vi "WILT Individual Plots.vi"(0 "File Name":T1, 1 "Station Data":T3 {"Night Cycle Count" format="%04d"; "Day Cycle Count" format="%04d"}, 2 "GUI Aisle 1 (SLAT).":T3[](array[typedef]) {"Night Cycle Count" format="%04d"; "Day Cycle Count" format="%04d"}, 5 "Error In":errorcluster, 6 "Station Index":i32) -> (14 "GUI Output":T3[](array[typedef]) {"Night Cycle Count" format="%04d"; "Day Cycle Count" format="%04d"}, 15 "Station Data Out":T3 {"Night Cycle Count" format="%04d"; "Day Cycle Count" format="%04d"}, 19 "Error Out":errorcluster)   [LabVIEW 2016]
uses:
  Type Definitions/WILT Dryer.ctl
  Type Definitions/WILT Dryer Details.ctl
  Type Definitions/WILT Agilent Channel Definition.ctl
  Type Definitions/WILT DAQ Data.ctl
  Utility/Save File/File Setup (Public)/Type Definition/Save File DOE File Path Control.ctl
  Utility/Save File/File Setup (Public)/Type Definition/Save File DOE Data Save Filepaths.ctl
  Utility/Save File/File Setup.lvlib
panel:
  in  "OK":bool
  out "Label":string
  in  "Tab Control":enum32{"Plots", "File Names", "Debug"}(tab)
  out "Mixed Signal Graph":cluster{timestamp[], "all rows":dbl[]}[](graph)
  in  "Debug":bool
  out "Lab ID":string
  out "Dryer Details.TR Number":string
  out "Day Cycle Count 2":i32
  out "Night Cycle Count 2":i32
  in  "Night Cycle Count":i32
  in  "Day Cycle Count":i32
  in  "TR Number:":string
  in  "Lab ID:":string
  # "Model Information"
  # "Day"
  # "Night"
  # "Day"
  # "Night"
  # "Day"
  # "Night"
  # "Day"
  # "Night"
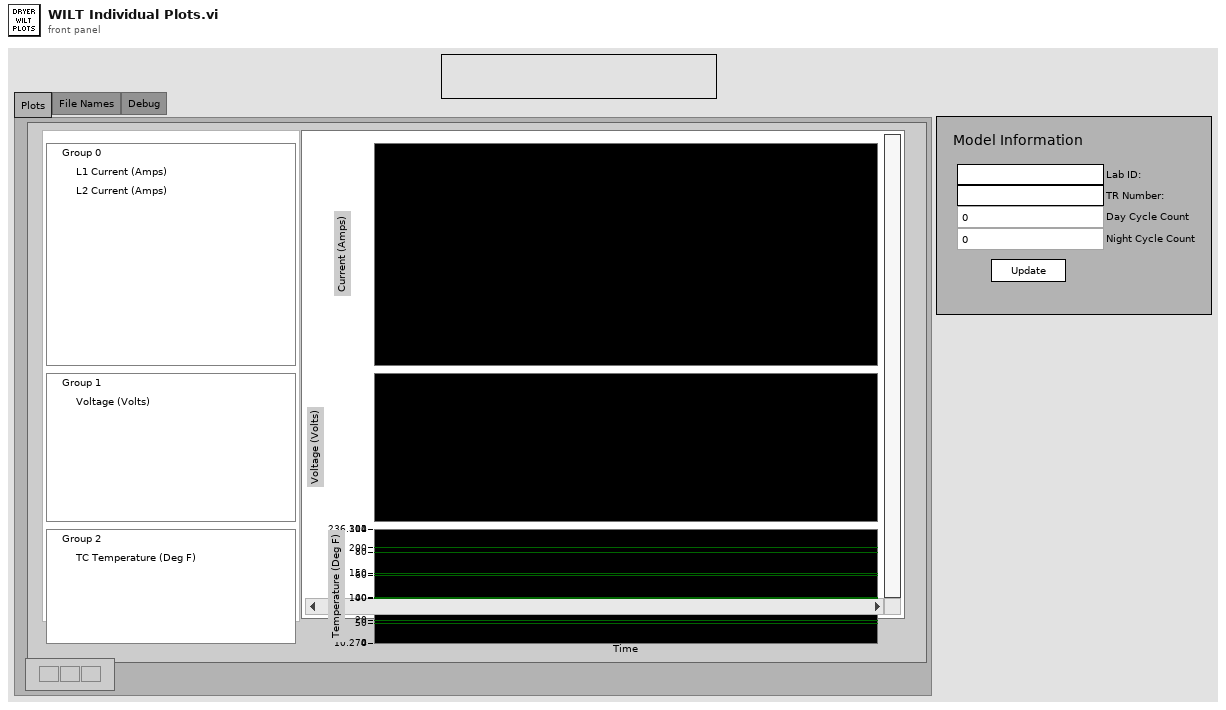
[diagram p1: front panel]
types:
  T1 = typedef "File Setup.lvlib/Save File DOE File Path Control.ctl" = cluster{"General Setup Paths":cluster{"Calibration File Path":path, "DOE Capacity Path":path, "Data Folder Path":path, "RLT Backup Data Path":path, "Tool Base Path":path, "General Startup Config Path":path, "File Save Previous Run Path":path, "File Save Configuration Data Path":path}, "Data File Paths":T2, "New Summary Created":bool, "Check Location Interval (Second)":i32}
  T2 = typedef "File Setup.lvlib/Save File DOE Data Save Filepaths.ctl" = cluster{"Data File Path":path, "Debug File Path":path, "Bus Log Path":path, "Current":path, "Summary":path}
  T3 = typedef "WILT Dryer.ctl" = cluster{"Lab ID":string, "Day Cycle Count":i32, "Station Label":string, "Dryer Details":T4, "Status Color":u32, "Invisible Button":bool, "Night Cycle Count":i32, "Station Index":i32, "Cycle Index":string, "Audit Alert":bool, "Agilent Channel Definition":T5, "DAQ Data":T6}
  T4 = typedef "WILT Dryer Details.ctl" = cluster{"Station":string, "Lab ID":string, "TR Number":string}
  T5 = typedef "WILT Agilent Channel Definition.ctl" = cluster{"Channel":string, "Station":string, "Label":string, "Agilent Station":string, "Data":dbl}
  T6 = typedef "WILT DAQ Data.ctl" = cluster{"L1 Current":dbl, "L2 Current":dbl, "Temperature  Deg F (TC)":dbl, "Volts":dbl, "Volts (208)":dbl, "SW (208)":dbl}
  T7 = enum32{"invalid app kind", "Development System", "Run Time System", "Student Edition", "Embedded LabVIEW", "Evaluation", "Custom"}
  T8 = enum32{"Invalid", "Standard", "Closed", "Hidden", "Minimized", "Maximized"}
  T9 = cluster{"Core":cluster{"Current VI Reference":refnum<vi>, "Close Panel on Exit?":bool}, "File Name":T1, "Station Data":T3, "GUI Aisle 1 (SLAT).":T3[]}
  T10 = cluster{"Current VI Reference":refnum<vi>, "Close Panel on Exit?":bool}
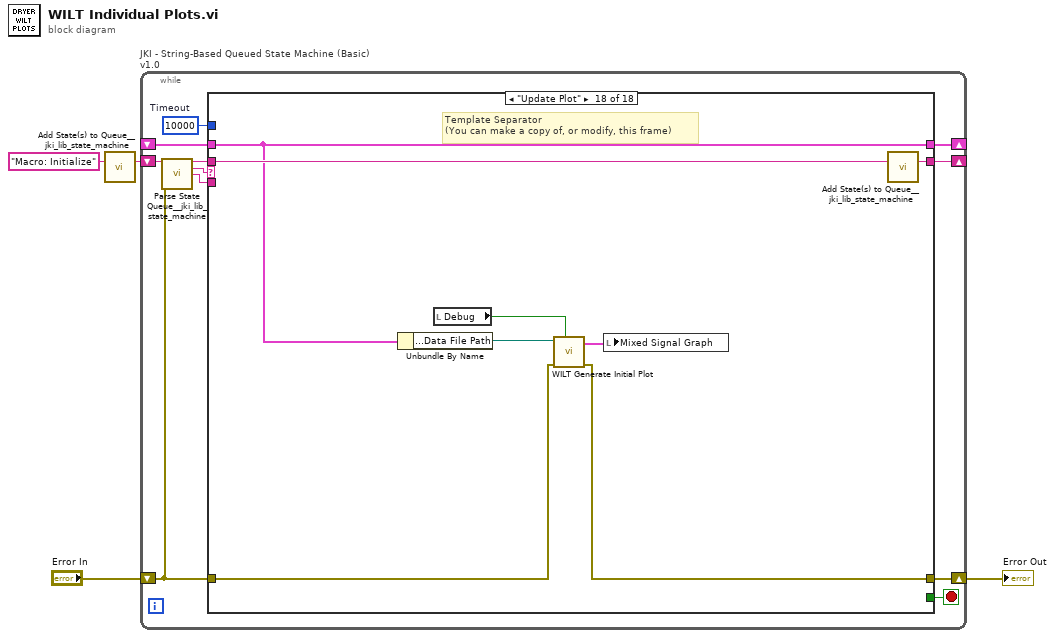
[diagram p0: block diagram]
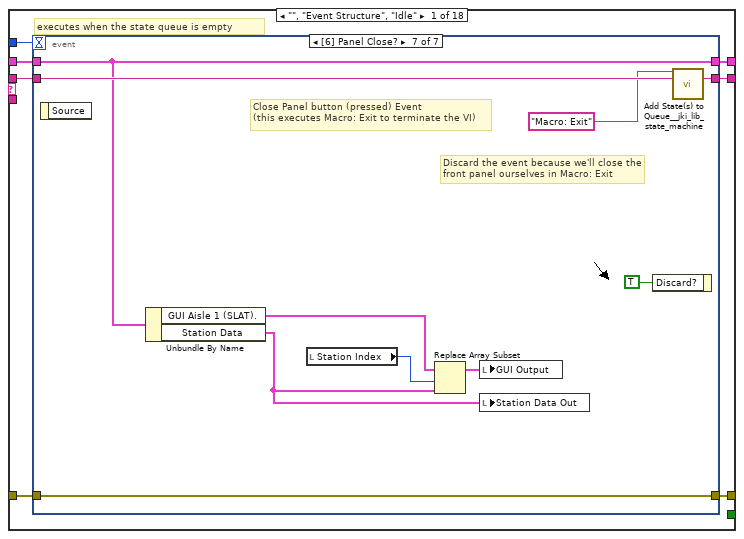
[diagram p2: hidden frame]
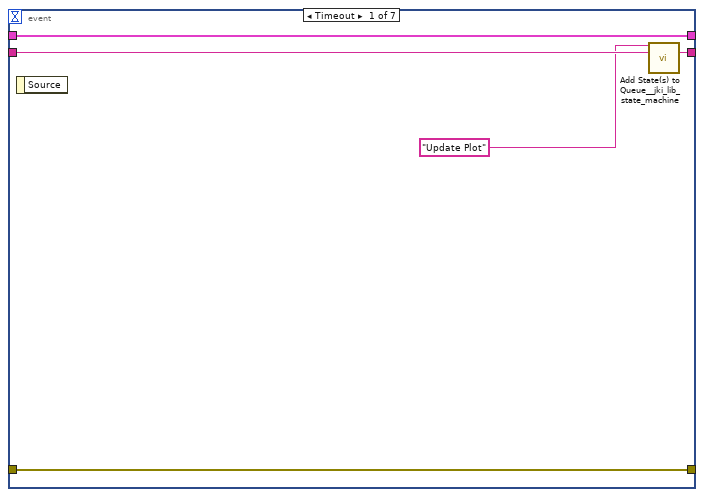
[diagram p3: hidden frame]
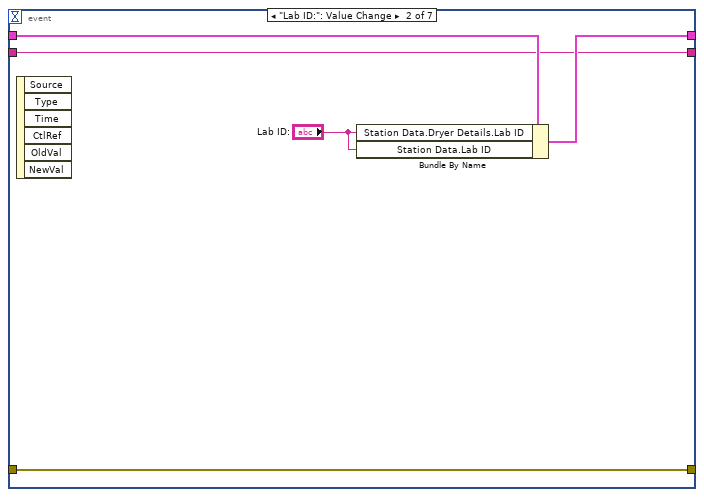
[diagram p4: hidden frame]
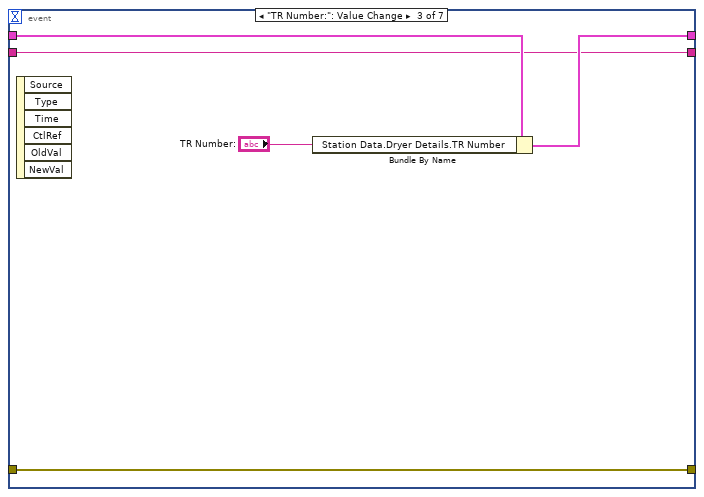
[diagram p5: hidden frame]
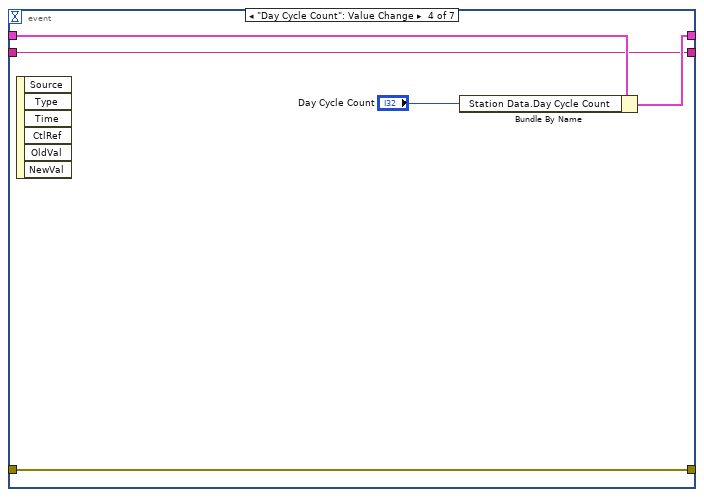
[diagram p6: hidden frame]
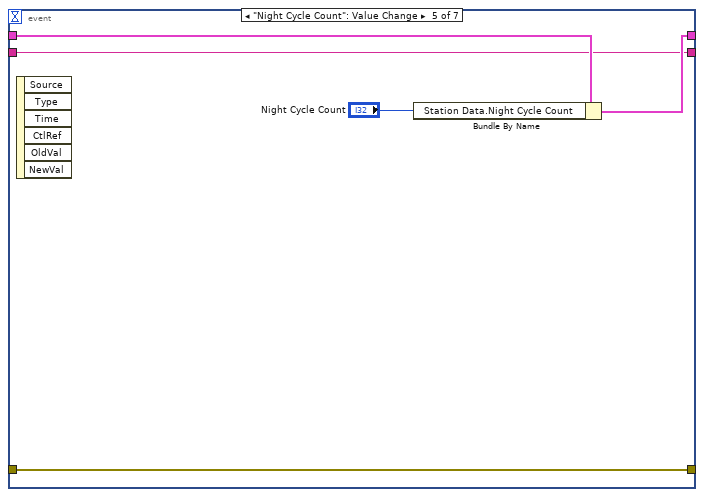
[diagram p7: hidden frame]
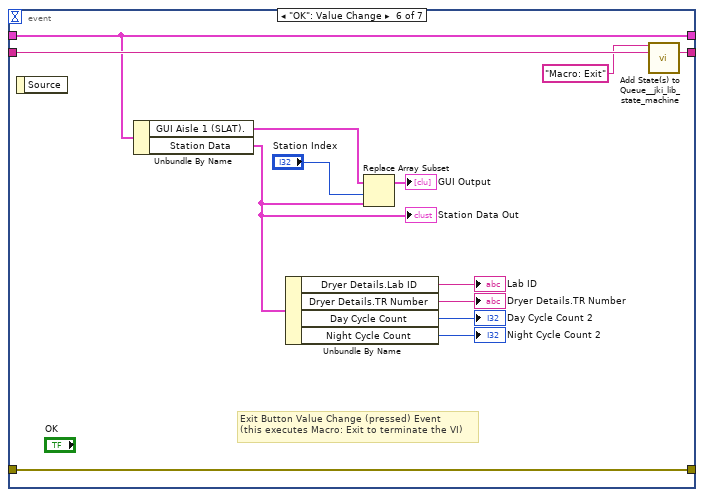
[diagram p8: hidden frame]
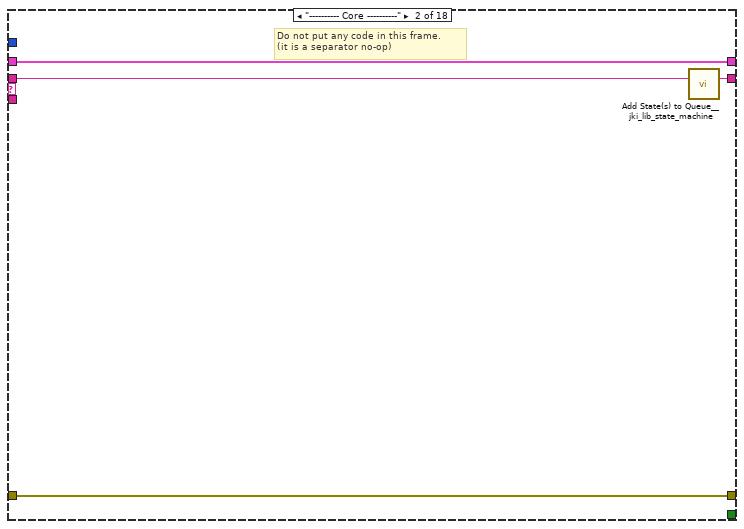
[diagram p9: hidden frame]
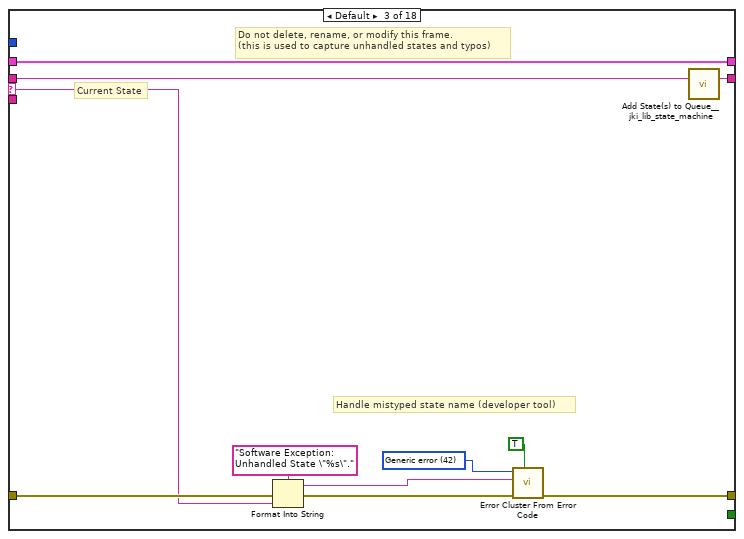
[diagram p10: hidden frame]
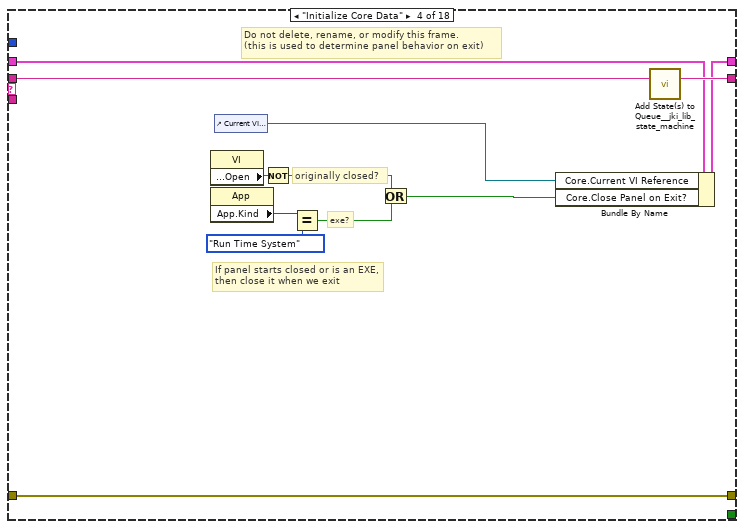
[diagram p11: hidden frame]
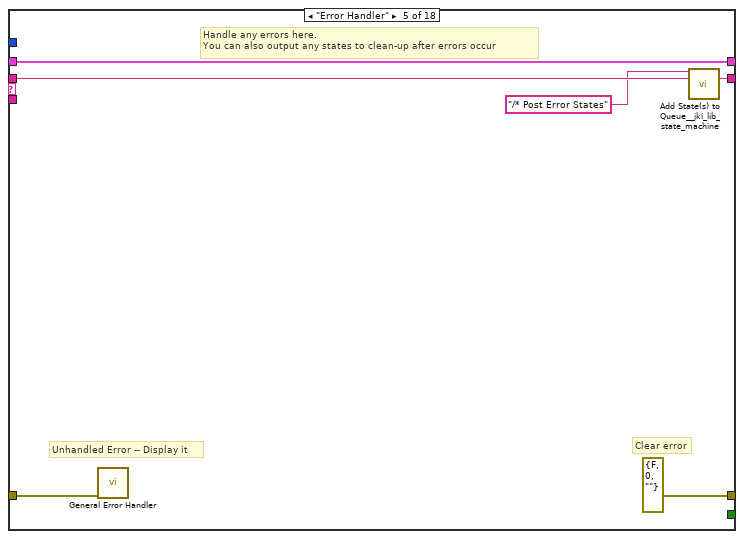
[diagram p12: hidden frame]
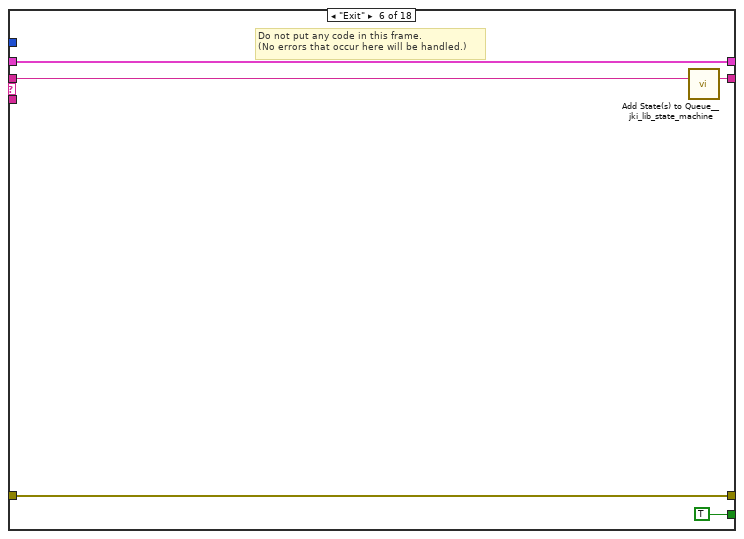
[diagram p13: hidden frame]
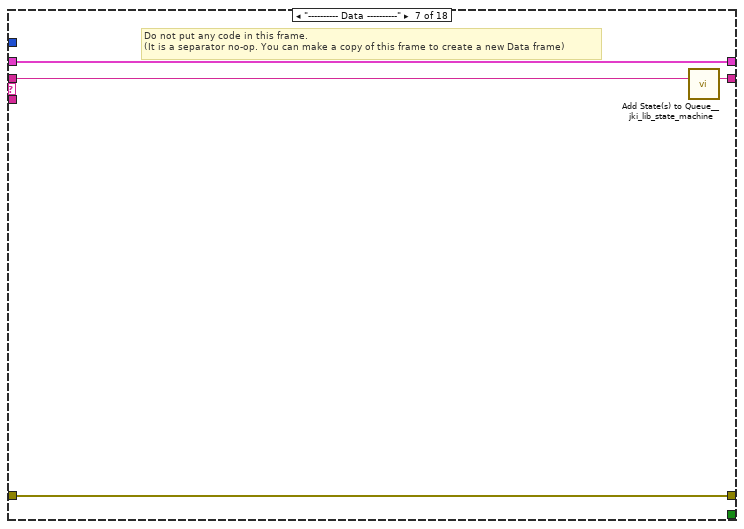
[diagram p14: hidden frame]
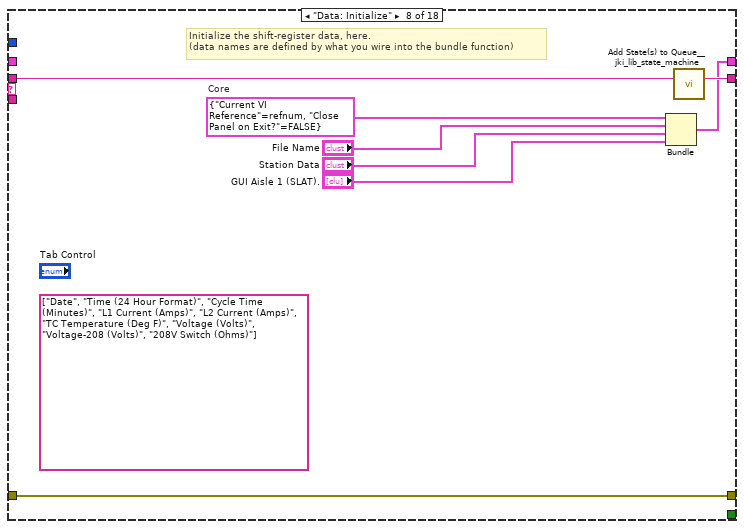
[diagram p15: hidden frame]
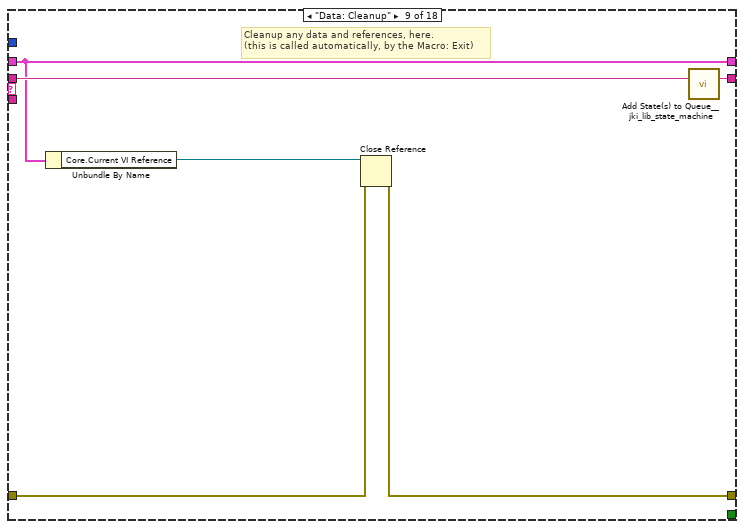
[diagram p16: hidden frame]
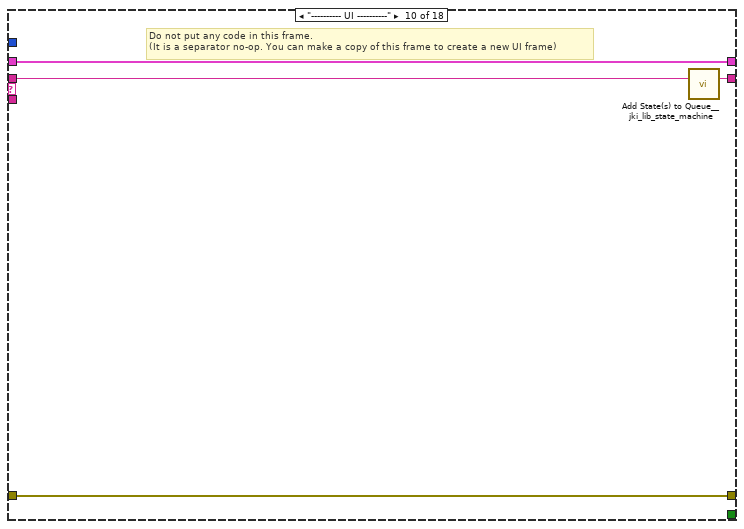
[diagram p17: hidden frame]
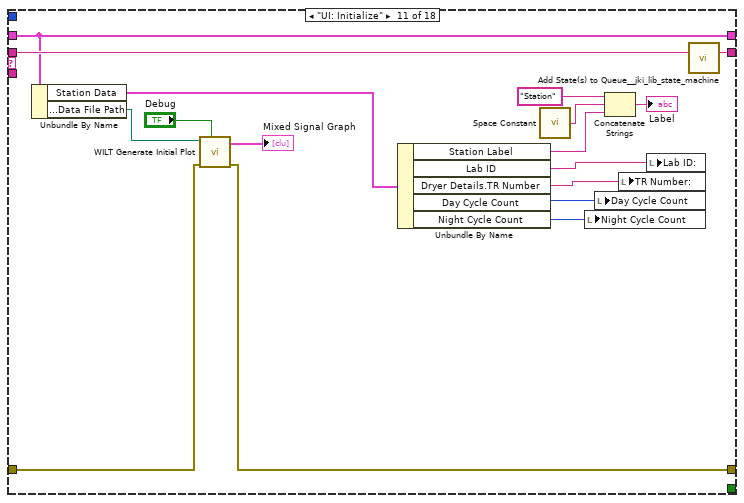
[diagram p18: hidden frame]
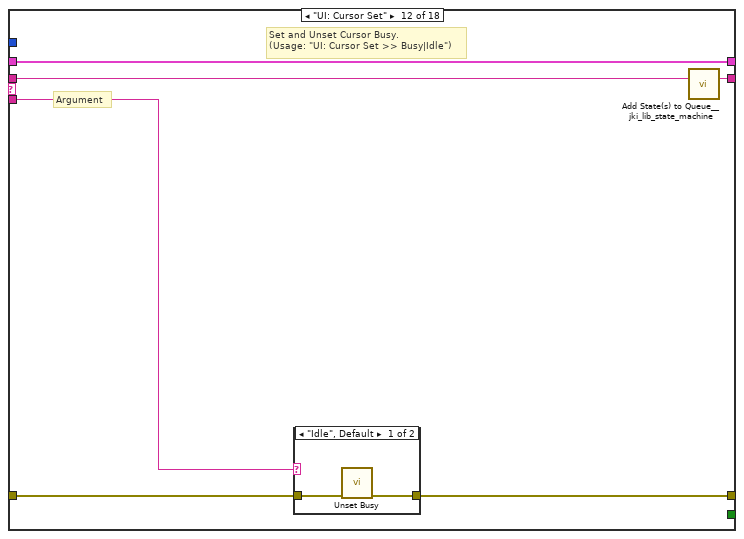
[diagram p19: hidden frame]
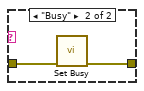
[diagram p20: hidden frame]
diagram:
  n1 = call <vilib>:"Add State(s) to Queue__jki_lib_state_machine.vi"("State(s) in (\"\")"="Macro: Initialize") -> ("States Out"=w4:string)  [unwired: 14 in]
  n2 = while "JKI - String-Based Queued State Machine (Basic) v1.0" {
    shift-right: [w8] -> _
    shift-left: _ -> [w7]
    shift-right: [w11] -> w2
    shift-left: "Error In" -> [w5]
    shift-right: [w10] -> _
    shift-left: w4 -> [w12]
    stop <- w9 stop-if-true
    w6 = 10000  # Timeout
    n3 = call <vilib>:"Parse State Queue__jki_lib_state_machine.vi"("State Queue"=w12, "Error In (no error)"=w5) -> ("Remaining States"=w14:string, "Current State"=w15:string, "Arguments"=w13:string)  [unwired: 11 in]
    n4 = case shown="\"Update Plot\"" w15 {
      selector: w15 -> [_ _ w75 _ _ _ _ _ _ _ _ _ _ _ _ _ _ _]
      tunnel: w14 -> [w22 w74 w79 w97 w103 w108 w112 w120 w126 w130 w147 w153 w164 w190 w195 w205 w209 w217]
      tunnel: w13 -> [_ _ _ _ _ _ _ _ _ _ _ w148 w158 _ _ _ _ _]
      tunnel: w7 -> [w20 w71 w77 w88 w100 w106 w109 _ w121 w127 w145 w151 w160 w187 w192 w202 w206 w214]
      tunnel: [w19 w72 w81 w94 errorcluster {"status"=FALSE, "code"=0, "source"=""} ("error out") w105 w110 w117 w122 w128 w141 w149 w161 w188 w193 w203 w207 w210] -> w11
      tunnel: w5 -> [w18 w72 w80 w94 w99 w105 w110 w117 w123 w128 w142 w150 w162 w188 w193 w203 w207 w211]
      tunnel: [w21 w73 w78 w96 w102 w107 w111 w119 w125 w129 w146 w152 w163 w189 w194 w204 w208 w216] -> w10
      tunnel: [_ _ _ _ _ TRUE _ _ _ _ _ _ _ _ _ _ _ _] -> w9
      tunnel: [w17 w71 w77 w95 w100 w106 w109 w118 w121 w127 w145 w151 w160 w187 w192 w202 w206 w214] -> w8
      tunnel: w6 -> [w16 _ _ _ _ _ _ _ _ _ _ _ _ _ _ _ _ _]
      frame "", "Event Structure", "Idle" {
        # "executes when the state queue is empty"
        n5 = event shown="[6] Panel Close?" {
          selector: _ -> [_ _ _ _ _ _ _]
          dyn-events: _ -> [_ _ _ _ _ _ _]
          timeout: w16 -> [_ _ _ _ _ _ _]
          tunnel: w22 -> [w27 w29 w35 w40 w45 w60 w70]
          tunnel: [w26 w29 w35 w40 w45 w59 w69] -> w21
          tunnel: w20 -> [w24 w31 w37 w42 w47 w53 w62]
          tunnel: [w25 w32 w34 w38 w43 w58 w68] -> w19
          tunnel: w18 -> [w25 w32 w34 w38 w43 w58 w68]
          tunnel: [w24 w30 w36 w41 w46 w53 w62] -> w17
          event Timeout {
            n6 = event-data() -> ()  [unwired: 1 in, 1 out]
            n7 = call <vilib>:"Add State(s) to Queue__jki_lib_state_machine.vi"("State(s) in Front (\"\")"="Update Plot" ("State(s) in Front (\"\")"), "State(s) in (\"\")"=w27) -> ("States Out"=w26:string)  [unwired: 13 in]
          }
          event "Lab ID:": Value Change {
            n8 = event-data() -> ()  [unwired: 1 in, 6 out]
            n9 = Bundle By Name(cluster=w31, "Station Data.Dryer Details.Lab ID"="Lab ID:", "Station Data.Lab ID"="Lab ID:") -> (w30:T9)
          }
          event "TR Number:": Value Change {
            n10 = event-data() -> ()  [unwired: 1 in, 6 out]
            n11 = Bundle By Name(cluster=w37, "Station Data.Dryer Details.TR Number"="TR Number:") -> (w36:T9)
          }
          event "Day Cycle Count": Value Change {
            n12 = event-data() -> ()  [unwired: 1 in, 6 out]
            n13 = Bundle By Name(cluster=w42, "Station Data.Day Cycle Count"="Day Cycle Count") -> (w41:T9)
          }
          event "Night Cycle Count": Value Change {
            n14 = event-data() -> ()  [unwired: 1 in, 6 out]
            n15 = Bundle By Name(cluster=w47, "Station Data.Night Cycle Count"="Night Cycle Count") -> (w46:T9)
          }
          event "OK": Value Change {
            # "Exit Button Value Change (pressed) Event\n(this executes Macro: Exit to terminate the VI)"
            n16 = event-data() -> ()  [unwired: 1 in, 1 out]
            n17 = Unbundle By Name(w53) -> ("GUI Aisle 1 (SLAT)."=w56:T3[], "Station Data"=w52:T3)
            "Station Data Out" <- w52
            n18 = Unbundle By Name(w52) -> ("Dryer Details.Lab ID"=→"Lab ID":string, "Dryer Details.TR Number"=→"Dryer Details.TR Number":string, "Day Cycle Count"=→"Day Cycle Count 2":i32, "Night Cycle Count"=→"Night Cycle Count 2":i32)
            n19 = Replace Array Subset(array=w56, new element=w52, index="Station Index") -> (→"GUI Output":T3[])
            n20 = call <vilib>:"Add State(s) to Queue__jki_lib_state_machine.vi"("State(s) in Front (\"\")"="Macro: Exit", "State(s) in (\"\")"=w60) -> ("States Out"=w59:string)  [unwired: 13 in]
          }
          event Panel Close? {
            # "Discard the event because we'll close the front panel ourselves in Macro: Exit"
            # "Close Panel button (pressed) Event\n(this executes Macro: Exit to terminate the VI)"
            n21 = event-data() -> ()  [unwired: 1 in, 1 out]
            n22 = Unbundle By Name(w62) -> ("GUI Aisle 1 (SLAT)."=w63:T3[], "Station Data"=w65:T3)
            n23 = local read "Station Index"() -> (w61:i32)
            n24 = Replace Array Subset(array=w63, new element=w65, index=w61) -> (w64:T3[])
            n25 = local write "GUI Output"(w64) -> ()
            n26 = local write "Station Data Out"(w65) -> ()
            n27 = event-data("Discard?"=TRUE) -> ()  [unwired: 1 in, 1 out]
            n28 = call <vilib>:"Add State(s) to Queue__jki_lib_state_machine.vi"("State(s) in Front (\"\")"="Macro: Exit", "State(s) in (\"\")"=w70) -> ("States Out"=w69:string)  [unwired: 13 in]
          }
        }
      }
      frame "---------- Core ----------" {
        # "Do not put any code in this frame.\n(it is a separator no-op)"
        n29 = call <vilib>:"Add State(s) to Queue__jki_lib_state_machine.vi"("State(s) in (\"\")"=w74) -> ("States Out"=w73:string)  [unwired: 14 in]
      }
      frame Default {
        w84 = 42 items=["No error", "Argument error", "Memory is full", "Out of zone", "End of file", "File already open", "Generic file I/O error", "File not found", "File permission error", "Disk is full", "Duplicate path", "Too many files open", "System feature not enabled", "Resource file not found", "Cannot add resource", "Resource not found", "Image not found", "Image memory error", "Pen does not exist", "Config type invalid", "Config token not found", "Config parse error", "Config memory error", "Bad external code format", "Bad external code offset", "External code not present", "Null window", "Destroy window error", "Null menu", "Print aborted", "Bad print record", "Print driver error", "Windows error during printing", "Memory error during printing", "Print dialog error", "Generic print error", "Invalid device refnum", "Device not found", "Device parameter error", "Device unit error", "Cannot open device", "Device call aborted", "Generic error", "Cancelled by user", "Object ID too low", "Object ID too high", "Object not in heap", "Unknown heap", "Unknown object (invalid DefProc)", "Unknown object (DefProc not in table)", "Message out of range", "Invalid (null) method", "Unknown message", "Manager call not supported", "Bad address", "Network operation in progress", "Network operation timed out", "Connection is busy", "Network attribute not supported", "Network error", "Address in use", "System out of memory", "Connection aborted", "Connection refused", "Not connected", "Already connected", "Connection closed", "Initialization error (interapplication manager)", "Bad occurrence", "Wait on unbound occurrence handler", "Occurrence queue overflow", "Datalog type conflict", "Unused", "Unrecognized type (interapplication manager)", "Memory corrupt", "Failed to make temporary DLL", "Old CIN version", "Drag socket not found", "Failed to load drop-object", "Failed to register OLE object", "Failed to release OLE object", "Format specifier type mismatch", "Unknown format specifier", "Too few format specifiers", "Too many format specifiers", "Scan failed", "Newer CIN version", "Error converting to variant", "Runtime menu error", "Password tampered", "Variant attribute not found", "Incompatible variant data type", "Event data is not available", "Event Store is not present", "Occurrence is not found", "Event Queue is not created", "Event info is not available", "Refnum passed is NULL", "Error retrieving Class GUID", "Error retrieving CoClass GUID", "Error retrieving TypeLib GUID.", "Bad built application magic bytes.", "Specific driver is different from the specific driver associated with the Logical Name.", "There is no session opened to the class driver.", "Max Error", "MAX - Error with config objects", "MAX - Error loading configuration", "MAX - Group not supported"]
        # "Current State"
        # "Do not delete, rename, or modify this frame.\n(this is used to capture unhandled states and typos)"
        # "Handle mistyped state name (developer tool)"
        n30 = Format Into String(format string="Software Exception: Unhandled State \"%s\"." ("message"), error in=w80, w75) -> (resulting string=w83:string, error out=w82:errorcluster)  [unwired: 1 in]
        n31 = call <vilib>:"Error Cluster From Error Code.vi"("show call chain? (False)"=TRUE, "error in (no error)"=w82, "error message (\"\")"=w83, "error code (0)"=w84) -> ("error out"=w81:errorcluster)  [unwired: 5 in]
        n32 = call <vilib>:"Add State(s) to Queue__jki_lib_state_machine.vi"("State(s) in (\"\")"=w79) -> ("States Out"=w78:string)  [unwired: 14 in]
      }
      frame "Initialize Core Data" {
        # "Do not delete, rename, or modify this frame.\n(this is used to determine panel behavior on exit)"
        # "originally closed?"
        # "exe?"
        # "If panel starts closed or is an EXE, then close it when we exit"
        n33 = property class="VI"() -> ("Front Panel.Open"=w93:bool)  [unwired: 2 in, 2 out]
        n34 = property class="App"() -> ("App.Kind"=w92:T7)  [unwired: 2 in, 2 out]
        n35 = control-ref of="Current VI Reference"() -> (w86:refnum<vi>)
        n36 = Not(x=w93) -> (.not. x?=w90:bool)
        n37 = Equal?(x=w92, y=T7."Run Time System" ("Application:Kind")) -> (x = y?=w89:bool)
        n38 = Or(x=w90, y=w89) -> (x .or. y?=w87:bool)
        n39 = Bundle By Name(cluster=w88, "Core.Current VI Reference"=w86, "Core.Close Panel on Exit?"=w87) -> (w95:T9)
        n40 = call <vilib>:"Add State(s) to Queue__jki_lib_state_machine.vi"("State(s) in (\"\")"=w97) -> ("States Out"=w96:string)  [unwired: 14 in]
      }
      frame "Error Handler" {
        # "Unhandled Error -- Display it"
        # "Handle any errors here.\nYou can also output any states to clean-up after errors occur"
        # "Clear error"
        n41 = call <vilib>:"General Error Handler.vi"("error in (no error)"=w99) -> ()  [unwired: 10 in, 5 out]
        n42 = call <vilib>:"Add State(s) to Queue__jki_lib_state_machine.vi"("State(s) in Front (\"\")"="/* Post Error States", "State(s) in (\"\")"=w103) -> ("States Out"=w102:string)  [unwired: 13 in]
      }
      frame "Exit" {
        # "Do not put any code in this frame.\n(No errors that occur here will be handled.)"
        n43 = call <vilib>:"Add State(s) to Queue__jki_lib_state_machine.vi"("State(s) in (\"\")"=w108) -> ("States Out"=w107:string)  [unwired: 14 in]
      }
      frame "---------- Data ----------" {
        # "Do not put any code in this frame.\n(It is a separator no-op. You can make a copy of this frame to create a new Data frame)"
        n44 = call <vilib>:"Add State(s) to Queue__jki_lib_state_machine.vi"("State(s) in (\"\")"=w112) -> ("States Out"=w111:string)  [unwired: 14 in]
      }
      frame "Data: Initialize" {
        (unwired) string[] ["Date", "Time (24 Hour Format)", "Cycle Time (Minutes)", "L1 Current (Amps)", "L2 Current (Amps)", "TC Temperature (Deg F)", "Voltage (Volts)", "Voltage-208 (Volts)", "208V Switch (Ohms)"] ("subarray")
        w116 = T10 {"Current VI Reference"=refnum, "Close Panel on Exit?"=FALSE}  # Core
        # "Initialize the shift-register data, here.\n(data names are defined by what you wire into the bundle function)"
        n45 = Bundle("Core"=w116, "File Name"="File Name", "Station Data"="Station Data", "GUI Aisle 1 (SLAT)."="GUI Aisle 1 (SLAT).") -> (w118:T9)  [unwired: 1 in]
        n46 = call <vilib>:"Add State(s) to Queue__jki_lib_state_machine.vi"("State(s) in (\"\")"=w120) -> ("States Out"=w119:string)  [unwired: 14 in]
      }
      frame "Data: Cleanup" {
        # "Cleanup any data and references, here.\n(this is called automatically, by the Macro: Exit)"
        n47 = Unbundle By Name(w121) -> ("Core.Current VI Reference"=w124:refnum<vi>)
        n48 = Close Reference(reference=w124, error in (no error)=w123) -> (error out=w122:errorcluster)
        n49 = call <vilib>:"Add State(s) to Queue__jki_lib_state_machine.vi"("State(s) in (\"\")"=w126) -> ("States Out"=w125:string)  [unwired: 14 in]
      }
      frame "---------- UI ----------" {
        # "Do not put any code in this frame.\n(It is a separator no-op. You can make a copy of this frame to create a new UI frame)"
        n50 = call <vilib>:"Add State(s) to Queue__jki_lib_state_machine.vi"("State(s) in (\"\")"=w130) -> ("States Out"=w129:string)  [unwired: 14 in]
      }
      frame "UI: Initialize" {
        n51 = Unbundle By Name(w145) -> ("Station Data"=w132:T3, "File Name.Data File Paths.Data File Path"=w144:path)
        n52 = call "WILT Generate Initial Plot.vi"("Debug"="Debug", "Error In"=w142, "Data File Path"=w144) -> ("Error Out"=w141:errorcluster, "Mixed Signal Graph"=→"Mixed Signal Graph":cluster{timestamp[], "all rows":dbl[]}[])  [unwired: 7 in]
        n53 = Unbundle By Name(w132) -> ("Station Label"=w136:string, "Lab ID"=w140:string, "Dryer Details.TR Number"=w137:string, "Day Cycle Count"=w139:i32, "Night Cycle Count"=w138:i32)
        n54 = call <vilib>:"Space Constant.vi"() -> ("String"=w134:string)
        n55 = local write "Night Cycle Count"(w138) -> ()
        n56 = local write "Day Cycle Count"(w139) -> ()
        n57 = Concatenate Strings("Station" ("string"), w134, w136) -> (→"Label":string)
        n58 = local write "TR Number:"(w137) -> ()
        n59 = local write "Lab ID:"(w140) -> ()
        n60 = call <vilib>:"Add State(s) to Queue__jki_lib_state_machine.vi"("State(s) in (\"\")"=w147) -> ("States Out"=w146:string)  [unwired: 14 in]
      }
      frame "UI: Cursor Set" {
        # "Argument"
        # "Set and Unset Cursor Busy.\n(Usage: \"UI: Cursor Set >> Busy|Idle\")"
        n61 = case shown="\"Idle\", Default" w148 {
          tunnel: w150 -> [w155 w157]
          tunnel: [w154 w156] -> w149
          frame "Idle", Default {
            n62 = call <vilib>:"Unset Busy.vi"("error in (no error)"=w155) -> ("error out"=w154:errorcluster)  [unwired: 10 in]
          }
          frame "Busy" {
            n63 = call <vilib>:"Set Busy.vi"("error in (no error)"=w157) -> ("error out"=w156:errorcluster)  [unwired: 9 in, 1 out]
          }
        }
        n64 = call <vilib>:"Add State(s) to Queue__jki_lib_state_machine.vi"("State(s) in (\"\")"=w153) -> ("States Out"=w152:string)  [unwired: 14 in]
      }
      frame "UI: Front Panel State" {
        # "Argument"
        # "Set Front Panel Open or Closed\n(Usage: \"UI: Front Panel State >> Open|Close\")"
        n65 = Unbundle By Name(w160) -> ("Core.Current VI Reference"=w159:refnum<vi>)
        n66 = case shown="\"Open\", Default" w158 {
          tunnel: w162 -> [w168 w181]
          tunnel: [w170 w182] -> w161
          tunnel: w159 -> [w169 w179]
          frame "Open", Default {
            n67 = property class="VI"(reference=w169, error in=w168) -> (reference out=w166:refnum<vi>, error out=w167:errorcluster, "Front Panel.Open"=w165:bool)
            n68 = case shown="False" w165 {
              tunnel: [w173 w176] -> w170
              tunnel: w167 -> [w172 w176]
              tunnel: w166 -> [w171 _]
              frame False {
                n69 = invoke class="VI" method="FP.Open"(reference=w171, error in=w172, "Activate"=TRUE, "State"=T8."Standard") -> (error out=w173:errorcluster)  [unwired: 1 in, 4 out]
              }
              frame True {
              }
            }
          }
          frame "Close" {
            n70 = property class="VI"(reference=w179, error in=w181) -> (reference out=w178:refnum<vi>, error out=w180:errorcluster, "Front Panel.Open"=w177:bool)
            n71 = case shown="True" w177 {
              tunnel: [w183 w186] -> w182
              tunnel: w180 -> [w183 w185]
              tunnel: w178 -> [_ w184]
              frame False {
              }
              frame True {
                n72 = invoke class="VI" method="FP.Close"(reference=w184, error in=w185) -> (error out=w186:errorcluster)  [unwired: 1 in, 2 out]
              }
            }
          }
        }
        n73 = call <vilib>:"Add State(s) to Queue__jki_lib_state_machine.vi"("State(s) in (\"\")"=w164) -> ("States Out"=w163:string)  [unwired: 14 in]
      }
      frame "---------- Macro ----------" {
        # "Do not put any code in this frame.\n(It is a separator no-op. You can make a copy of this frame to create a new Macro frame)"
        n74 = call <vilib>:"Add State(s) to Queue__jki_lib_state_machine.vi"("State(s) in (\"\")"=w190) -> ("States Out"=w189:string)  [unwired: 14 in]
      }
      frame "Macro: Initialize" {
        w191 = "Data: Initialize\nInitialize Core Data\nUI: Initialize\nUI: Front Panel State >> Open"  # Data: Initialize Initialize Core Data UI: Initialize UI: Front Panel State >> Open
        # "Initialization Macro\n(This is called once, when the VI starts)"
        n75 = call <vilib>:"Add State(s) to Queue__jki_lib_state_machine.vi"("State(s) in Front (\"\")"=w191, "State(s) in (\"\")"=w195) -> ("States Out"=w194:string)  [unwired: 13 in]
      }
      frame "Macro: Exit" {
        # "Exit Macro\n(This is called once, when the VI exits)"
        n76 = Unbundle By Name(w202) -> ("Core.Close Panel on Exit?"=w201:bool)
        n77 = Select(t="UI: Front Panel State >> Close", s=w201, f="") -> (s? t:f=w198:string)
        n78 = call <vilib>:"Add State(s) to Queue__jki_lib_state_machine.vi"("State(s) in (\"\")"=w198, "State(s) at Back (\"\")"="Data: Cleanup\nExit") -> ("States Out"=w196:string)  [unwired: 13 in]
        n79 = call <vilib>:"Add State(s) to Queue__jki_lib_state_machine.vi"("State(s) in Front (\"\")"=w196, "State(s) in (\"\")"=w205) -> ("States Out"=w204:string)  [unwired: 13 in]
      }
      frame "---------- New Category ----------" {
        # "Template Separator\n(You can make a copy of, or modify, this frame)"
        n80 = call <vilib>:"Add State(s) to Queue__jki_lib_state_machine.vi"("State(s) in (\"\")"=w209) -> ("States Out"=w208:string)  [unwired: 14 in]
      }
      frame "Update Plot" {
        # "Template Separator\n(You can make a copy of, or modify, this frame)"
        n81 = Unbundle By Name(w214) -> ("File Name.Data File Paths.Data File Path"=w215:path)
        n82 = local read "Debug"() -> (w212:bool)
        n83 = call "WILT Generate Initial Plot.vi"("Debug"=w212, "Error In"=w211, "Data File Path"=w215) -> ("Error Out"=w210:errorcluster, "Mixed Signal Graph"=w213:cluster{timestamp[], "all rows":dbl[]}[])  [unwired: 7 in]
        n84 = local write "Mixed Signal Graph"(w213) -> ()
        n85 = call <vilib>:"Add State(s) to Queue__jki_lib_state_machine.vi"("State(s) in (\"\")"=w217) -> ("States Out"=w216:string)  [unwired: 14 in]
      }
    }
  }
  "Error Out" <- w2
